vi "rwr_Set Voltage Range.vi"(4 "Show in Debugger?":bool=TRUE, 6 "Message Priority":T1=enum."Normal", 7 "Caller in":refnum<class "Worker.lvclass">, 8 "error in":errorcluster, 9 "timeout (ms)":i32=5000, 10 "Data in":T3, 11 "Fluke DMM in":refnum<class "Fluke DMM.lvclass">) -> (0 "error out":errorcluster, 2 "Reply Data out":T2, 3 "dup Fluke DMM out":refnum<class "Fluke DMM.lvclass">)   [LabVIEW 2020, in "Fluke DMM.lvclass"]
doc: "This VI sends a <b>Public API Request with Reply</b> message to an MHL case of the Worker that owns this VI. This VI will wait until it receives a <b>Reply</b> message back from the Worker that owns this VI. If the wait time exceeds <b>timeout (ms)</b>, an error will be returned.\n---\nSet the voltage range of the DMM."
uses:
  Fluke DMM.lvclass
  C:/Program Files (x86)/National Instruments/LabVIEW 2020/vi.lib/addons/_Workers/Library/Classes/Worker/Worker.lvclass
  <vilib>/addons/_Workers/Library/Classes/Worker/Worker.lvclass
  Interface 1/rwr_Set Voltage Range.ctl
  Interface 1/rwr_Set Voltage Range Reply.ctl
  <vilib>/addons/_Workers/Library/Classes/Message/Priority.ctl
  <vilib>/addons/_Workers/Library/Case Label.ctl
  <vilib>/addons/_Workers/Library/Classes/Message Queue/Message Queue.lvclass
  <vilib>/addons/_Workers/Library/Workers.lvlib
  <vilib>/addons/_Workers/Library/Classes/Message/Message.lvclass
  Interface 1/Interface 1.lvclass
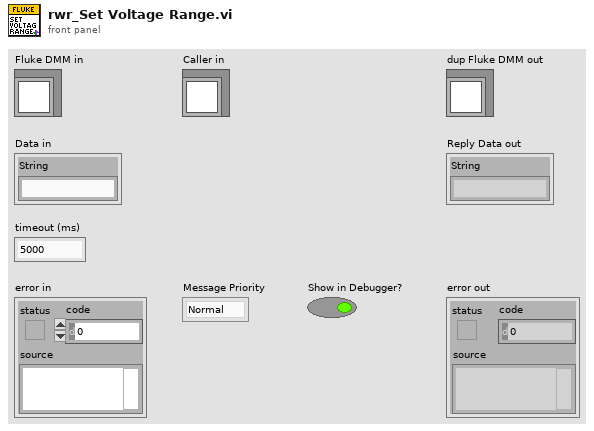
[diagram p1: front panel]
types:
  T1 = typedef "Workers.lvlib/Message.lvclass/Priority.ctl" = enum16{"Low", "Normal", "High"}
  T2 = typedef "Interface 1.lvclass/rwr_Set Voltage Range Reply.ctl" = cluster{"String":string}
  T3 = typedef "Interface 1.lvclass/rwr_Set Voltage Range.ctl" = cluster{"String":string}
  T4 = typedef "Workers.lvlib/Case Label.ctl" = string
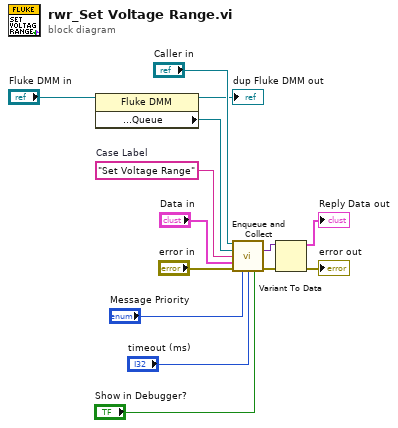
[diagram p0: block diagram]
diagram:
  w14 = T4 "Set Voltage Range"  # Case Label
  n1 = property class="Fluke DMM"(reference="Fluke DMM in") -> (reference out=→"dup Fluke DMM out":refnum<class "Fluke DMM.lvclass">, "Accessors:Read:Public API:Queue"=w13:refnum<class "Message Queue.lvclass">)  [unwired: 1 in, 1 out]
  n2 = call-dynamic "Enqueue and Collect.vi"("Worker"="Caller in", "Message Queue"=w13, "Case Label"=w14, "Data"="Data in", "error in (no error)"="error in", "Priority (Normal)"="Message Priority", "timeout in ms"="timeout (ms)", "Send Message to Debugger? (T)"="Show in Debugger?") -> ("Data out"=w12:variant, "error out"=w11:errorcluster)  [unwired: 4 in, 2 out]
  n3 = Variant To Data(error in=w11, Variant=w12) -> (data=→"Reply Data out":T2, error out=→"error out":errorcluster)  [unwired: 1 in]
